vi "LastLoadedFile.vi"(0 "SetFileLocation":refnum<vi>, 1 "Last Loaded File":refnum<vi>, 4 "GUIName":string, 5 "DIMControSet in":refnum<vi>[](array[refnum]), 6 "SetValueInfo in":refnum<vi>[](array[refnum]), 7 "NewVal":T1, 9 "ListOfBases_Data":refnum<vi>) -> ()   [LabVIEW 2014, in "Panels.lvlib"]
uses:
  Panels.lvlib
  CSlibraries-extern/DimLVEvent/DimIndicators/DimIndicators.anyType.ctl
  CSlibraries/UtilityLib/UtilityLib.valueStatus.ctl
  CS_Core/CSSystem/CoreLib/CoreLib.lvlib
  CSlibraries/UtilityLib/UtilityLib.lvlib
  CSlibraries-extern/DimLVEvent/DimIndicators/DimIndicators.lvlib
panel:
  in  "ListOfBases_Data":T1={"data"="NOLINK", "no link"=TRUE, "quality"=-1, "timeStamp"=0.0}
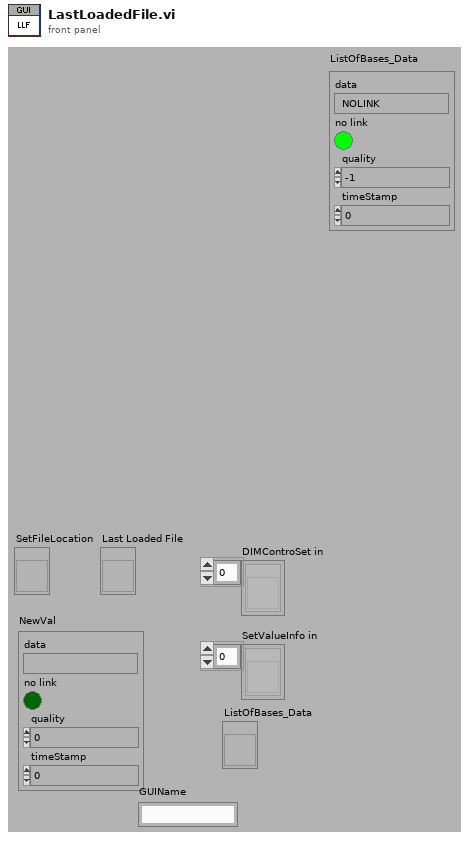
[diagram p1: front panel]
types:
  T1 = typedef "DimIndicators.lvlib/DimIndicators.anyType.ctl" = cluster{"data":string, "no link":bool, "quality":i32, "timeStamp":dbl}
  T2 = typedef "UtilityLib.lvlib/UtilityLib.valueStatus.ctl" = enum16{"no info available", "stand by/off", "on", "warning", "alarm/malfunction", "not implemented", "user action required", "important information", "system default", "control default", "indicator default", "button default"}
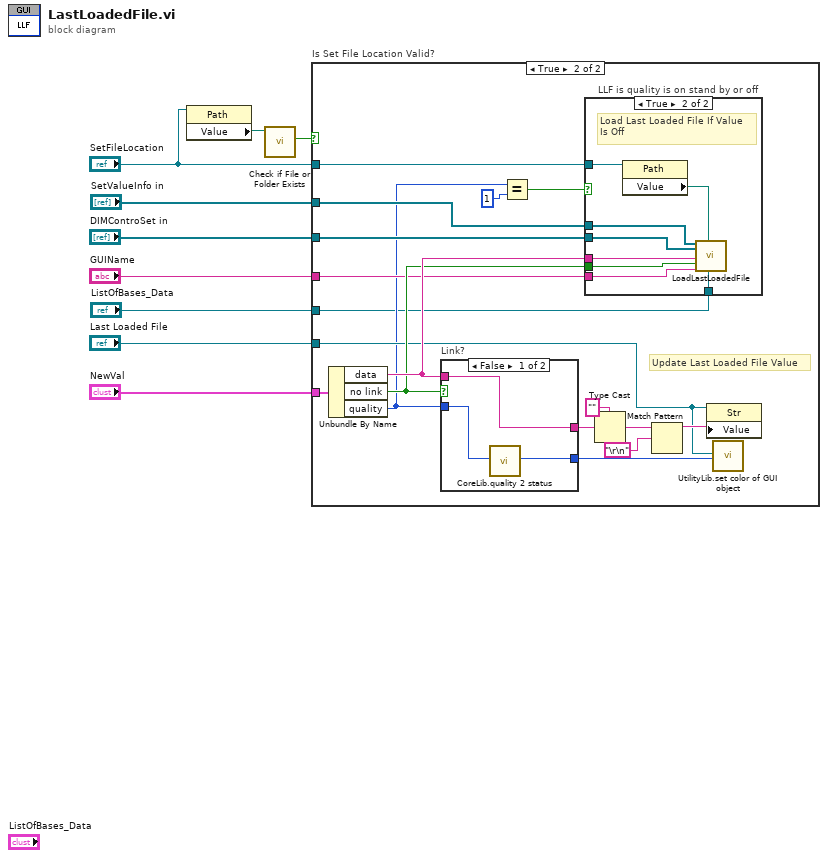
[diagram p0: block diagram]
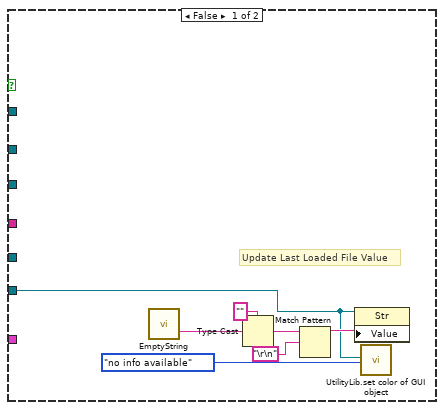
[diagram p2: hidden frame]
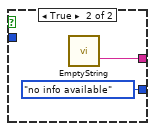
[diagram p4: hidden frame]
diagram:
  n1 = property class="Path"(reference="SetFileLocation") -> ("Value"=w5:path)  [unwired: 1 in, 2 out]
  n2 = call <vilib>:"Check if File or Folder Exists.vi"("path"=w5) -> ("file or folder exists?"=w6:bool)  [unwired: 8 in, 2 out]
  n3 = case "Is Set File Location Valid?" shown="True" w6 {
    tunnel: "NewVal" -> [_ w34]
    tunnel: "DIMControSet in" -> [_ w31]
    tunnel: "SetFileLocation" -> [_ w23]
    tunnel: "Last Loaded File" -> [w10 w22]
    tunnel: "GUIName" -> [_ w21]
    tunnel: "SetValueInfo in" -> [_ w20]
    tunnel: "ListOfBases_Data" -> [_ w17]
    frame False {
      # "Update Last Loaded File Value"
      n4 = call "EmptyString.vi"() -> ("String"=w12:string)
      n5 = Type Cast(type="" ("regular expression"), x=w12) -> (*(type *) &x=w13:string)
      n6 = Match Pattern(string=w13, regular expression="\r\n") -> (before substring=w11:string)  [unwired: 1 in, 3 out]
      n7 = property class="Str"(reference=w10, "Value"=w11) -> ()  [unwired: 1 in, 2 out]
      n8 = call "UtilityLib.set color of GUI object.vi"("GUI object Ref"=w10, "valueStatus"=UtilityLib.valueStatus."no info available") -> ()  [unwired: 17 in, 1 out]
    }
    frame True {
      # "Update Last Loaded File Value"
      n9 = Unbundle By Name(w34) -> ("data"=w32:string, "no link"=w30:bool, "quality"=w19:i32)
      n10 = case "Link?" shown="False" w30 {
        tunnel: w19 -> [w45 _]
        tunnel: [w44 UtilityLib.valueStatus."no info available" ("valueStatus")] -> w33
        tunnel: w32 -> [w43 _]
        tunnel: [w43 w46] -> w25
        frame False {
          n11 = call "CoreLib.quality 2 status.vi"("quality"=w45) -> ("valueStatus"=w44:T2)  [unwired: 18 in]
        }
        frame True {
          n12 = call "EmptyString.vi"() -> ("String"=w46:string)
        }
      }
      n13 = Equal?(x=w19, y=1 ("x")) -> (x = y?=w29:bool)
      n14 = case "LLF is quality is on stand by or off" shown="True" w29 {
        tunnel: w32 -> [_ w41]
        tunnel: w30 -> [_ w37]
        tunnel: w31 -> [_ w40]
        tunnel: w23 -> [_ w39]
        tunnel: w21 -> [_ w38]
        tunnel: w20 -> [_ w36]
        tunnel: w17 -> [_ w35]
        frame False {
        }
        frame True {
          # "Load Last Loaded File If Value\nIs Off"
          n15 = property on="Property Node" class="Path"(reference=w39) -> ("Value"=w42:path)  [unwired: 1 in, 2 out]
          n16 = call "LoadLastLoadedFile.vi"("SetValueInfo in"=w36, "DIMControSet in"=w40, "Data"=w41, "No Link?"=w37, "GUIName"=w38, "PanelLocation"=w42, "ListOfBases_Data"=w35) -> ()  [unwired: 12 in, 1 out]
        }
      }
      n17 = Type Cast(type="" ("regular expression"), x=w25) -> (*(type *) &x=w26:string)
      n18 = Match Pattern(string=w26, regular expression="\r\n") -> (before substring=w24:string)  [unwired: 1 in, 3 out]
      n19 = property class="Str"(reference=w22, "Value"=w24) -> ()  [unwired: 1 in, 2 out]
      n20 = call "UtilityLib.set color of GUI object.vi"("GUI object Ref"=w22, "valueStatus"=w33) -> ()  [unwired: 17 in, 1 out]
    }
  }
